vi "Create Box Plot.vi"(6 "target image filepath":path, 8 "error in (no error)":errorcluster, 9 "labels":T1, 10 "datasets":dbl[][](array[numeric])) -> (0 "error out":errorcluster, 2 "boxplot":picture)   [LabVIEW 2019, in "Python Visualizations.lvlib"]
uses:
  plot_labels.ctl
  <vilib>/Utility/sysdir.llb/System Directory Type.ctl
  Python Visualizations.lvlib
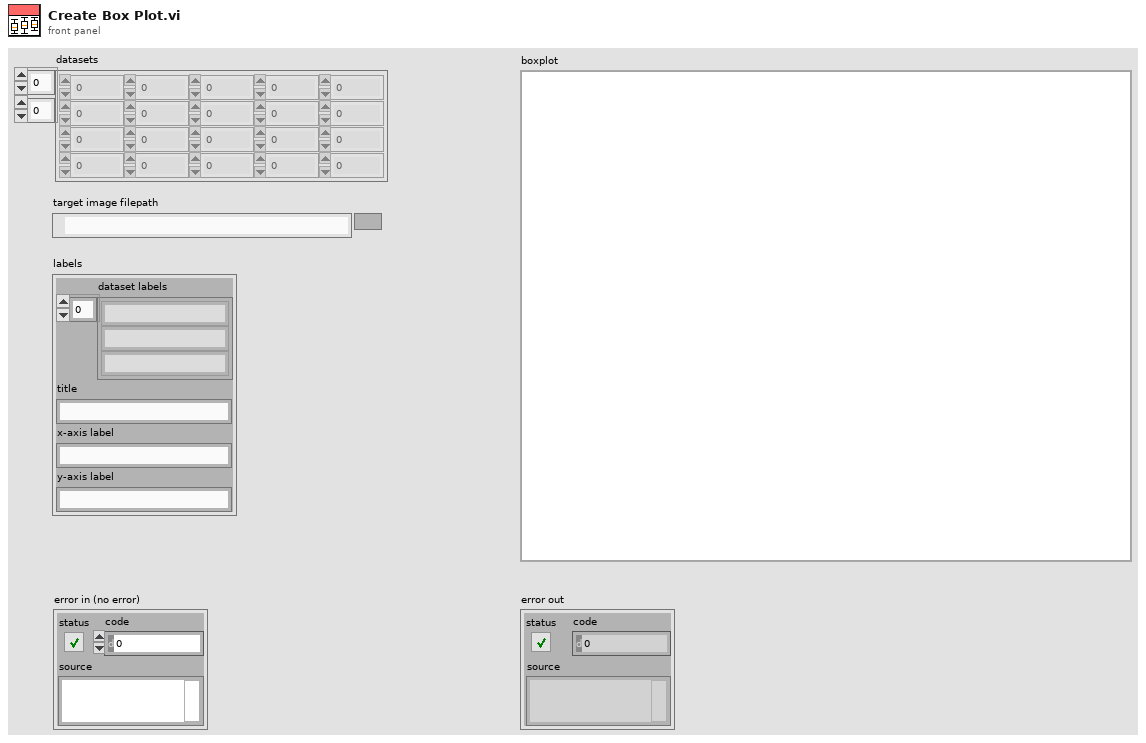
[diagram p1: front panel]
types:
  T1 = typedef "Python Visualizations.lvlib/plot_labels.ctl" = cluster{"dataset labels":string[], "title":string, "x-axis label":string, "y-axis label":string}
  T2 = typedef "System Directory Type.ctl" = i32
  T3 = typedef "imagedata.ctl" = cluster{"image type":i32, "image depth":i32, "image":u8[], "mask":u8[], "colors":u32[], "Rectangle":cluster{"left":i16, "top":i16, "right":i16, "bottom":i16}}
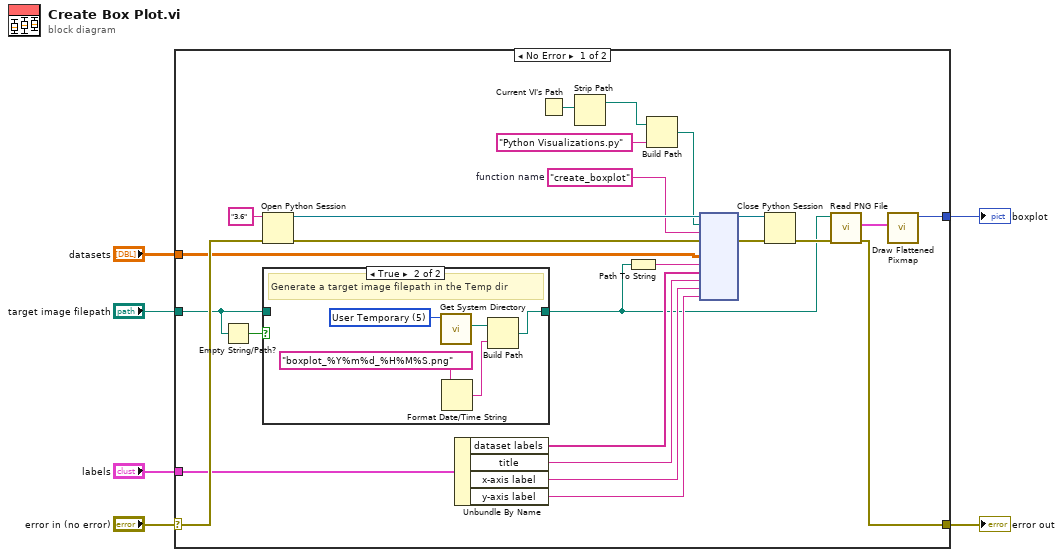
[diagram p0: block diagram]
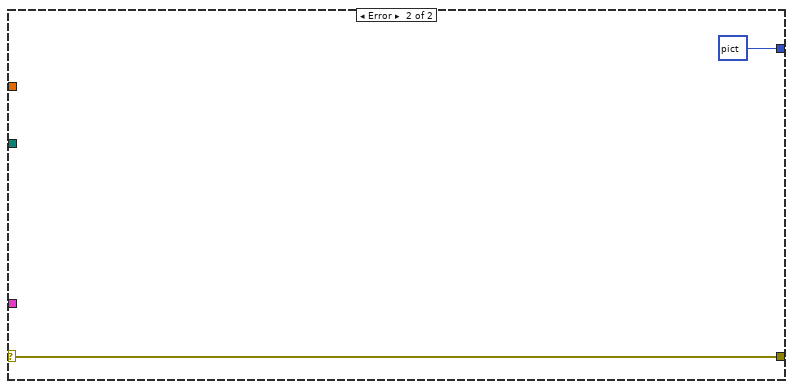
[diagram p3: hidden frame]
diagram:
  n1 = case shown="No Error" "error in (no error)" {
    selector: "error in (no error)" -> [w20 w39]
    tunnel: [w22 picture data[5B] ("new picture")] -> w6
    tunnel: [w19 w39] -> w4
    tunnel: "labels" -> [w15 _]
    tunnel: "target image filepath" -> [w9 _]
    tunnel: "datasets" -> [w7 _]
    frame No Error {
      w26 = "create_boxplot"  # function name
      n2 = Empty String/Path?(string/path=w9) -> (empty?=w10:bool)
      n3 = Open Python Session(python version="3.6" ("Python version"), 3:w20) -> (session out=w31:refnum<k35>, error out=w29:errorcluster)  [unwired: 1 in]
      n4 = case shown="True" w10 {
        tunnel: w9 -> [w32 _]
        tunnel: [w32 w33] -> w8
        frame False {
          # "Caller has specified a target image filepath"
        }
        frame True {
          w37 = T2 5 items=["User Home"=0, "User Desktop"=1, "User Documents"=2, "User Application Data"=3, "User Preferences"=4, "User Temporary"=5, "Public Documents"=6, "Public Application Data"=7, "Public Preferences"=8, "Public Cache"=13, "System Core Libraries"=9, "System Installed Libraries"=10, "Application Files"=11, "Boot Volume Root"=12] ("system directory type")
          # "Generate a target image filepath in the Temp dir"
          n5 = call <vilib>:"Get System Directory.vi"("system directory type"=w37) -> ("system directory"=w36:path)  [unwired: 10 in]
          n6 = Format Date/Time String(time format string (%c)="boxplot_%Y%m%d_%H%M%S.png") -> (date/time string=w34:string)  [unwired: 2 in]
          n7 = Build Path(base path=w36, name or relative path=w34) -> (appended path=w33:path)
        }
      }
      n8 = Unbundle By Name(w15) -> ("dataset labels"=w14:string[], "title"=w13:string, "x-axis label"=w12:string, "y-axis label"=w11:string)
      n9 = Current VI's Path() -> (path=w17:path)
      n10 = Strip Path(path=w17) -> (stripped path=w16:path)  [unwired: 1 out]
      n11 = Path To String(path=w8) -> (string=w30:string)
      n12 = Build Path(base path=w16, name or relative path="Python Visualizations.py") -> (appended path=w27:path)
      n13 = node(w31, w27, w26, w29, w7, w30, w14, w13, w12, w11) -> (w25:refnum<k35>, w24:errorcluster)  [unwired: 8 in, 2 out]
      n14 = Close Python Session(session in=w25, error in=w24) -> (11:w21:errorcluster)
      n15 = call <vilib>:"Read PNG File.vi"("error in (no error)"=w21, "path to PNG file"=w8) -> ("error out"=w19:errorcluster, "image data"=w23:T3)  [unwired: 7 in, 1 out]
      n16 = call <vilib>:"Draw Flattened Pixmap.vi"("image data"=w23) -> ("new picture"=w22:picture)  [unwired: 8 in]
    }
    frame Error {
    }
  }
  "error out" <- w4
  "boxplot" <- w6
